vi "Read U16 1D Value.vi"(8 "error in (no error)":errorcluster, 11 "Double Float in":refnum<class "Abs_U32 Integer 1D.lvclass">) -> (0 "error out":errorcluster, 2 "U16":u16[](array[numeric]), 3 "Double Float out":refnum<class "Abs_U32 Integer 1D.lvclass">)   [LabVIEW 2021, in "Abs_U32 Integer 1D.lvclass"]
uses:
  Abs_U32 Integer 1D.lvclass
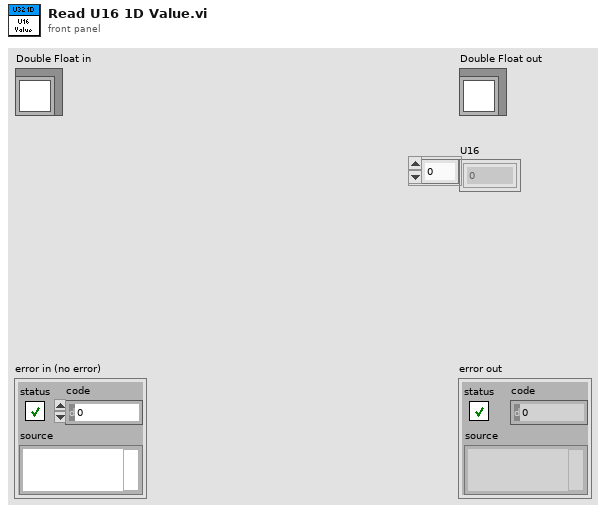
[diagram p1: front panel]
types:
  T1 = typedef "Abs_U32 Integer 1D.lvclass/Type.ctl" = u32[]
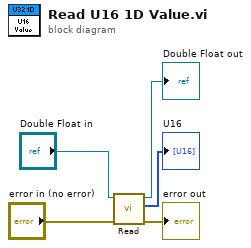
[diagram p0: block diagram]
diagram:
  n1 = call-dynamic "Read.vi"("error in (no error)"="error in (no error)", "Double Float.lvclass_340760 in"="Double Float in") -> ("error out"=→"error out":errorcluster, "Value"=→"U16":T1, "Double Float.lvclass_340760 out"=→"Double Float out":refnum<class "Abs_U32 Integer 1D.lvclass">)  [unwired: 7 in]
